vi "Type_1.vi"(7 "프런트패널 윈도우:동작":T2(ring)=enum."Default", 8 "에러 입력":errorcluster caption="에러 입력(에러 없음)", 11 "세부분류코드":string caption="확장자없는 파일 이름") -> (0 "error out":errorcluster)   [LabVIEW 2020]
uses:
  Support/Controls/Cmd_Mouse Popup.ctl
  Support/Controls/Clst_Query Info.ctl
  Support/Controls/Cmd_Read Query.ctl
  Support/Public/Polymorph/Data Class_2D Str.vi
  Support/Public/Polymorph/Array Dedup_1D Str.vi
  Support/Public/Polymorph/Cell Space_Table.vi
  <vilib>/addons/database/NI_Database_API.lvlib
panel:
  in  "탭 컨트롤":enum32{"검색", "등록", "CMC"}(tab)
  out "Calfunc":string[][](array[string])
  in  "Procedure 검색":T1(tab)
  in  "OPT_CODE 1":string(combo) caption="옵션 선택"
  in  "Func CbBox 1":string(combo) caption="Length_5"
  in  "Model List 1":i32(listbox) caption="모델 및 옵션 리스트"
  out "Load Proc 1":string[][](table) caption="등록된 교정 Procedure"
  in  "OPT_CODE 2":string(combo) caption="옵션 선택"
  in  "Func CbBox 2":string(combo) caption="Angle_1"
  in  "Model List 2":i32(listbox) caption="모델 및 옵션 리스트"
  out "Load Proc 2":string[][](table) caption="등록된 교정 Procedure"
  in  "OPT_CODE 3":string(combo) caption="옵션 선택"
  in  "Func CbBox 3":string(combo) caption="Magnification_1"
  in  "Model List 3":i32(listbox) caption="모델 및 옵션 리스트"
  out "Load Proc 3":string[][](table) caption="등록된 교정 Procedure"
  in  "OPT_CODE 4":string(combo) caption="옵션 선택"
  in  "Func CbBox 4":string(combo) caption="Right Angle_1"
  in  "Model List 4":i32(listbox) caption="모델 및 옵션 리스트"
  out "Load Proc 4":string[][](table) caption="등록된 교정 Procedure"
  in  "OPT_CODE 5":string(combo) caption="옵션 선택"
  in  "Func CbBox 5":string(combo) caption="AC Current Meter"
  in  "Model List 5":i32(listbox) caption="모델 및 옵션 리스트"
  out "Load Proc 5":string[][](table) caption="등록된 교정 Procedure"
  in  "OPT_CODE 6":string(combo) caption="옵션 선택"
  in  "Func CbBox 6":string(combo) caption="Frequency Meter"
  in  "Model List 6":i32(listbox) caption="모델 및 옵션 리스트"
  out "Load Proc 6":string[][](table) caption="등록된 교정 Procedure"
  in  "추가 버튼":bool
  out "소분류코드":string
  out "측정기명":string
  in  "단위":string(combo)
  in  "교정점 추가 버튼":bool
  in  "추가교정점":string
  out "Func_ext ?":bool
  out "배열":u32[](array[numeric])
  in  "Display 변경":bool
  in  "표시방식":string(combo)
  in  "Range":string(combo)
  in  "등록 버튼":bool
  in  "분해능 변경 버튼":bool
  in  "Proc":string[][](table) caption="등록할 교정 Procedure"
  in  "형식":string
  in  "옵션":string
  in  "분해능":string(combo)
  in  "교정기능":string(combo)
  out "CMC":string[][](table)
  # "항목정보"
  # "분해능 변경"
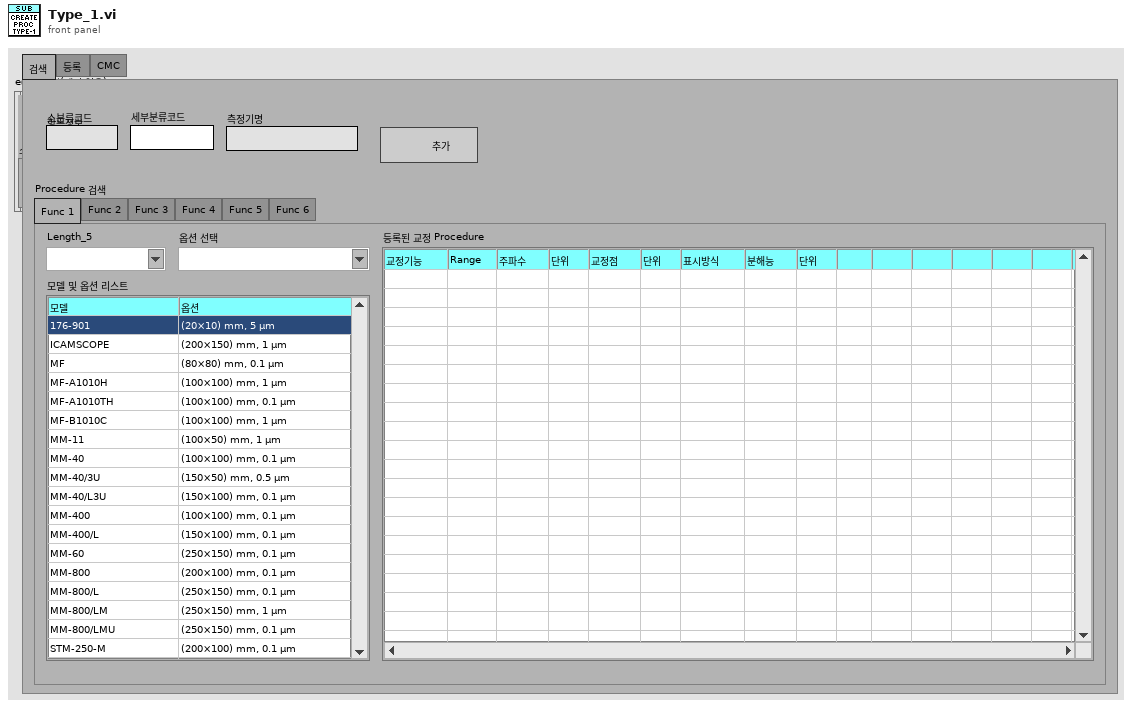
[diagram p1: front panel]
types:
  T1 = enum32{"Func 1", "Func 2", "Func 3", "Func 4", "Func 5", "Func 6"}
  T2 = enum32{"Invalid", "Default", "Floating", "Floating/Auto-Hide", "Modal"}
  T3 = typedef "Cmd_Mouse Popup.ctl" = enum16{"활성화", "메뉴선택"}
  T4 = cluster{"Shift":bool, "Ctrl":bool, "Alt":bool, "Cmd":bool, "Opt":bool}
  T5 = typedef "Clst_Query Info.ctl" = cluster{"사번":string, "등록번호":string, "업체명":string, "세부분류코드":string, "형식":string, "기기번호":string, "FUNC":string, "FUNC_EXT":string, "옵션":string, "추가문자열":string, "일자":string, "배열 1":string[], "배열 2":string[], "항목명":string, "문자열":string, "이름":string}
  T6 = typedef "Cmd_Read Query.ctl" = enum16{"교정자 이름 얻기", "인증교정자 얻기", "기술책임자 얻기", "기책부책 얻기", "등록번호 얻기", "등록정보 얻기", "업체정보 얻기", "교정일자(CAMAS) 얻기", "교정일자(CALSTD) 얻기", "교정환경 얻기", "교정절차서 목록 얻기", "교정절차서명 얻기", "교정절차 목록얻기", "교정절차 얻기", "PROC 교정절차 얻기", "PROC SPEC 얻기", "교정절차(Func별) 얻기", "교정절차(Func_ext별) 얻기", "기관코드 얻기", "교정기능(세부분류) 얻기", "교정기능(모델) 얻기", "교정기능 목록 얻기", "교정기능 명칭 얻기", "교정기능 항목명칭 얻기", "DB (사용기준기) 얻기", "DB (기준기이름) 얻기", "DB (기준기이름목록) 얻기", "DB (기준기목록) 얻기", "DB (기준기값) 얻기", "DB (CMC) 얻기", "DB (FUNC) 얻기", "DB (CALNAME) 얻기", "DB (STDNAME) 얻기", "DB (SPEC) 얻기", "모델(항목전체) 얻기", "모델(최대범위) 얻기", "모델(최소범위) 얻기", "모델(최대최소) 얻기", "모델(범위조건) 얻기", "모델(등록요청) 얻기", "모델(형식별) 얻기", "모델(조건별) 얻기", "모델(모델검색) 얻기", "세부분류 목록 얻기", "기준기등록리스트 얻기", "STD Cal Date Check", "DB등록일자 얻기", "적용항목 얻기", "기타정보 얻기", "기준기요청 얻기", "서버버전 얻기"}
  T7 = typedef "NI_Database_API.lvlib/Conn ObjectReference.ctl" = refnum<k1>
  T8 = typedef "LVRowAndColumnTypeDef.ctl" = cluster{"Row":i32, "Column":i32}
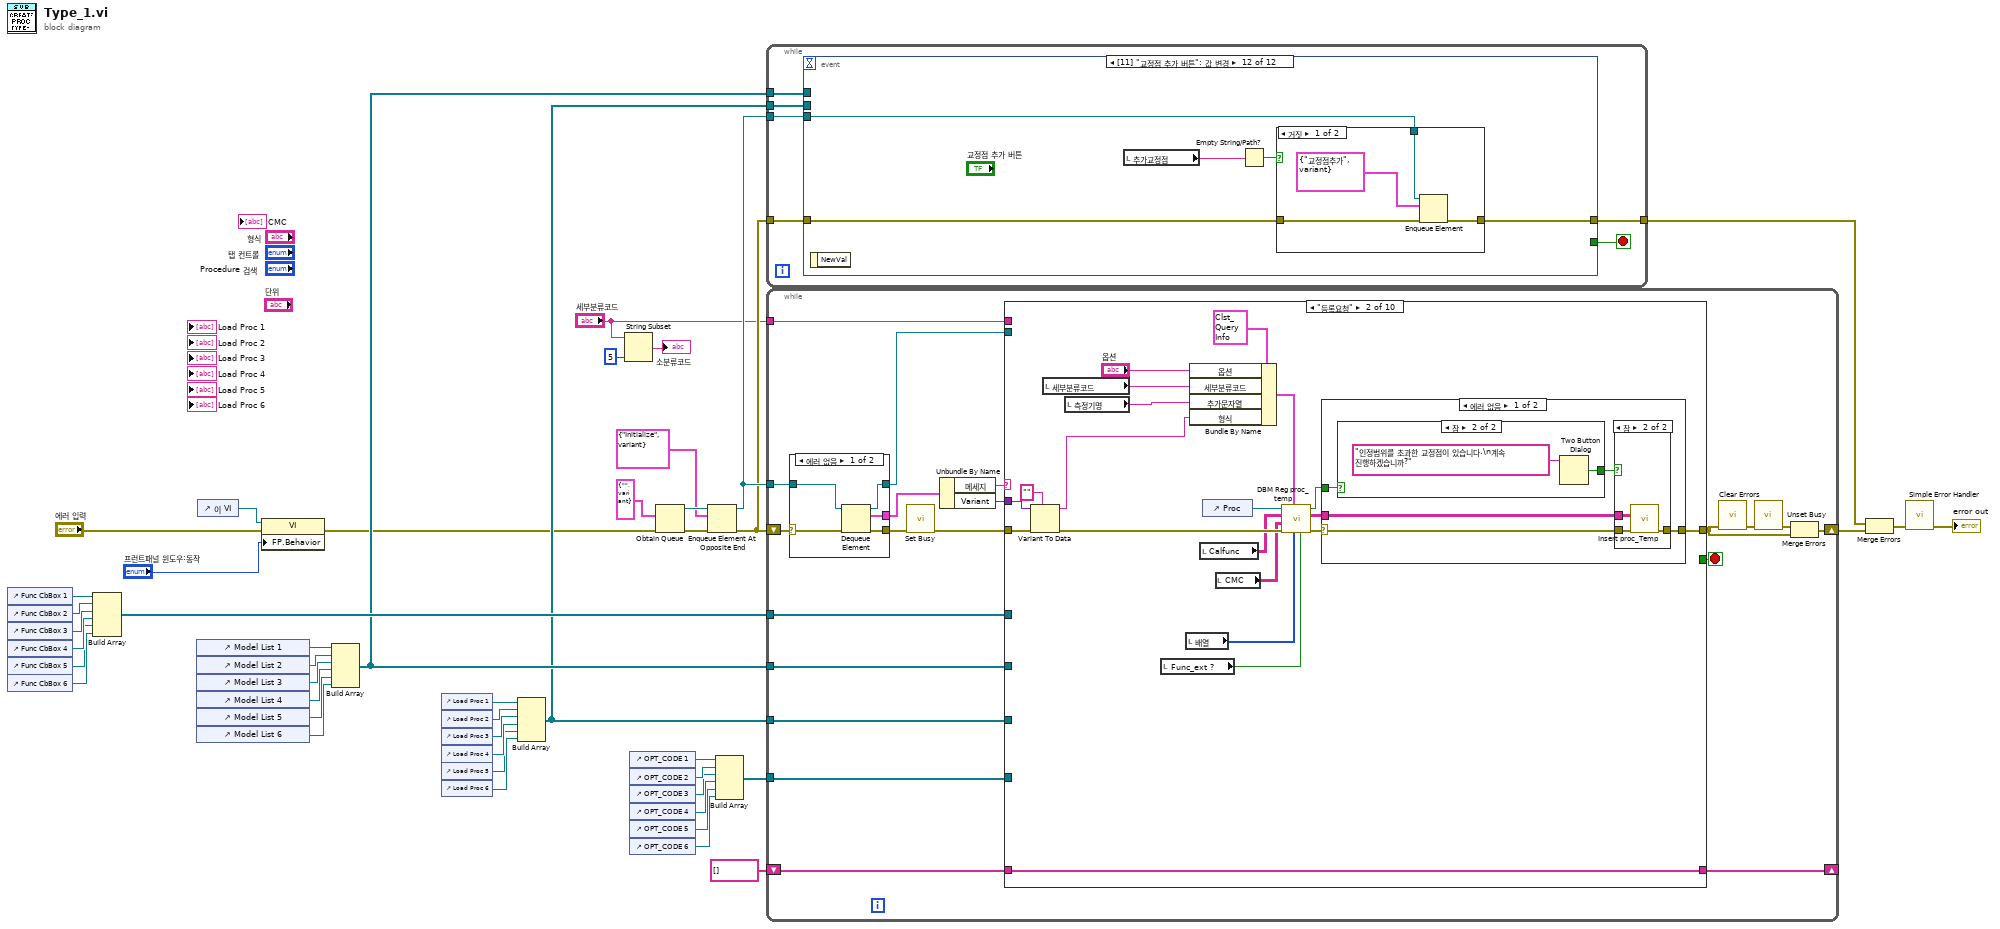
[diagram p0: block diagram]
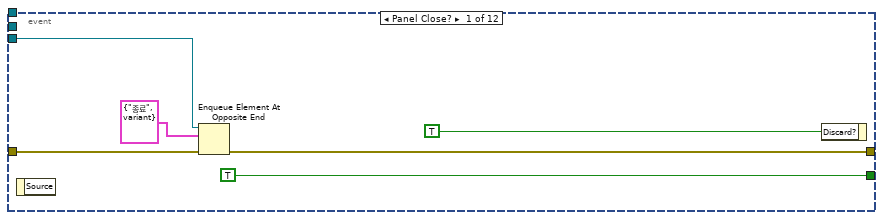
[diagram p2: hidden frame]
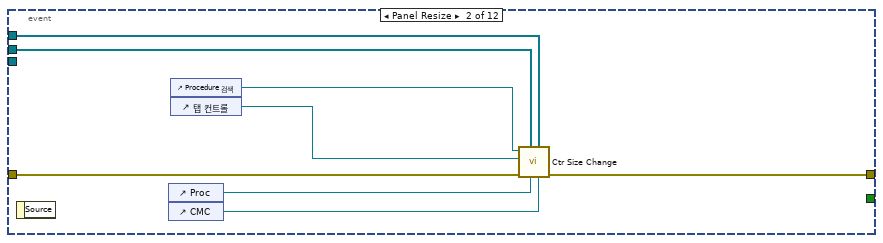
[diagram p3: hidden frame]
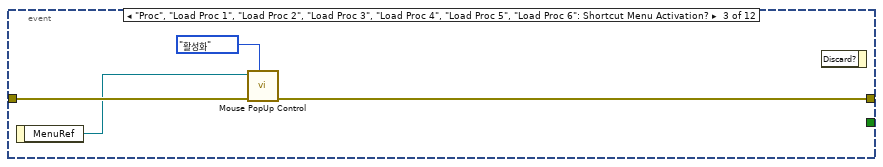
[diagram p4: hidden frame]
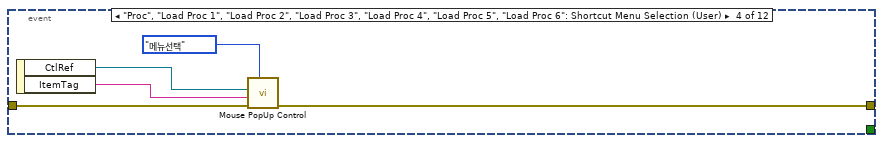
[diagram p5: hidden frame]
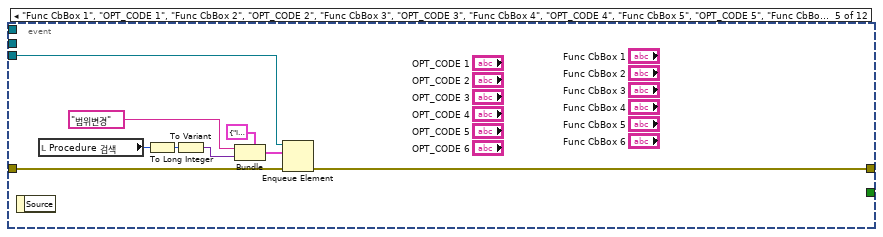
[diagram p6: hidden frame]
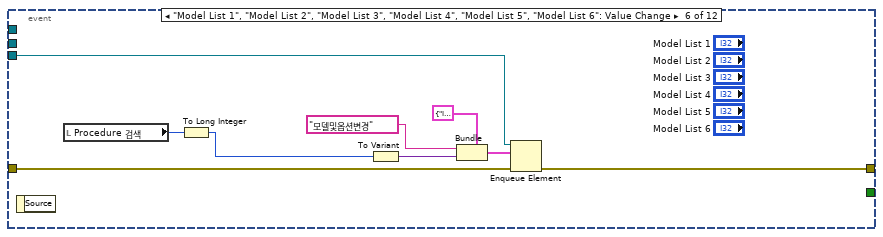
[diagram p7: hidden frame]
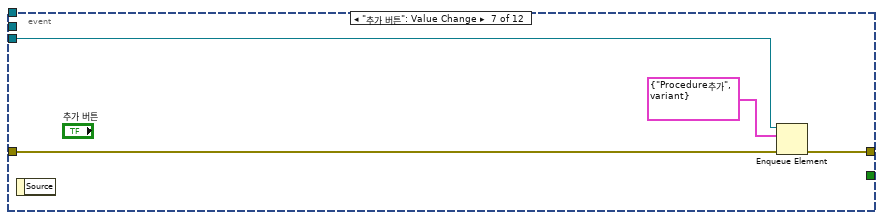
[diagram p8: hidden frame]
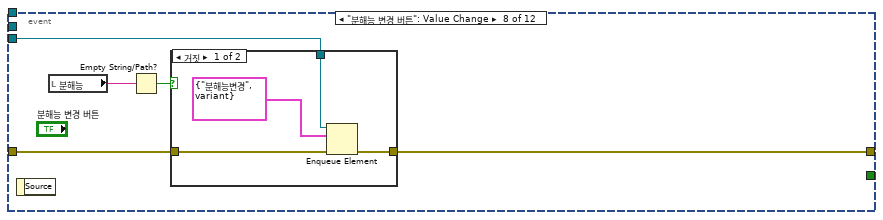
[diagram p9: hidden frame]
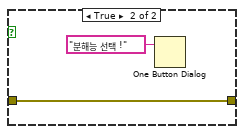
[diagram p10: hidden frame]
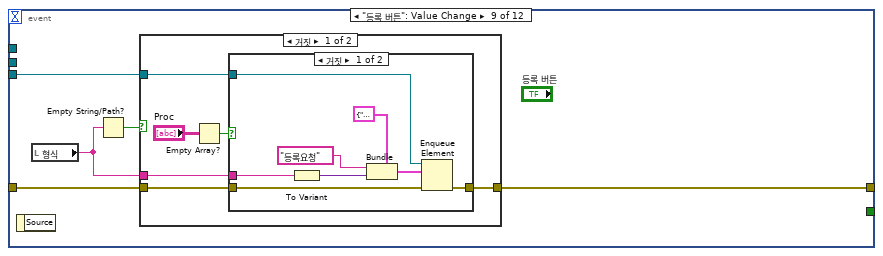
[diagram p11: hidden frame]
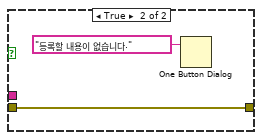
[diagram p12: hidden frame]
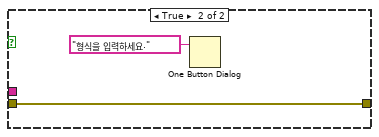
[diagram p13: hidden frame]
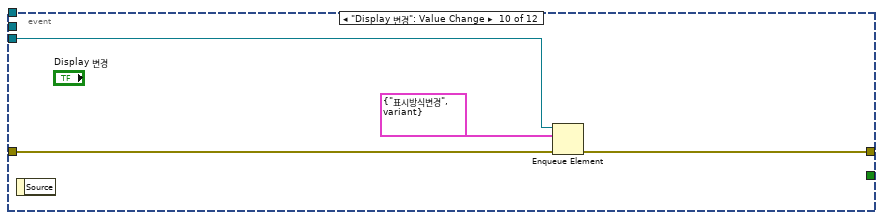
[diagram p14: hidden frame]
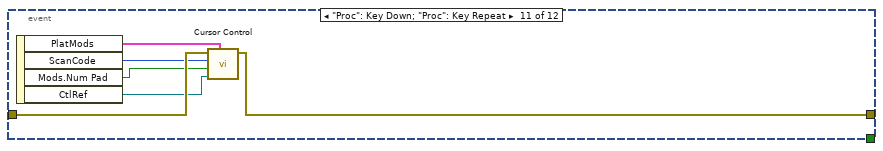
[diagram p15: hidden frame]
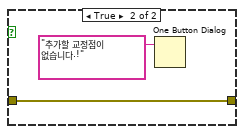
[diagram p16: hidden frame]
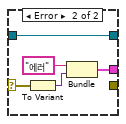
[diagram p17: hidden frame]
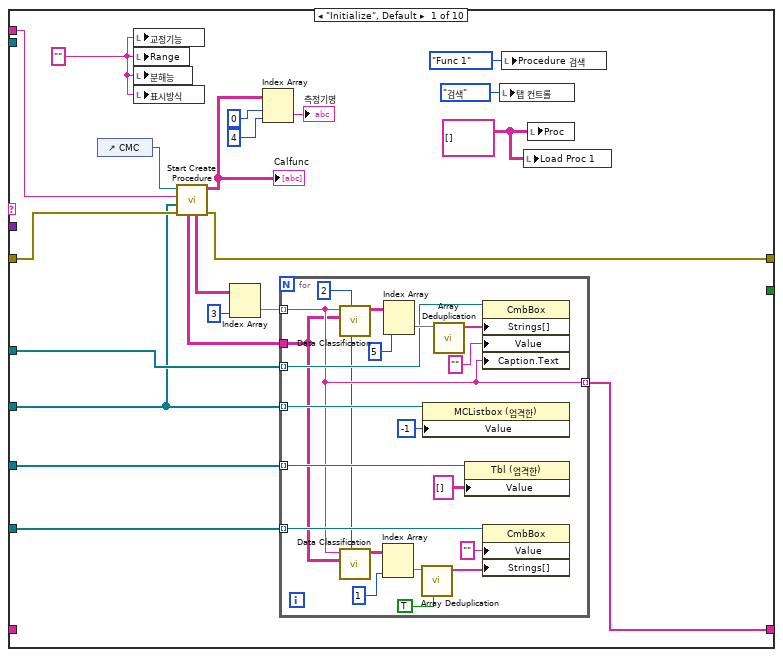
[diagram p18: hidden frame]
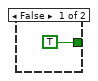
[diagram p19: hidden frame]
diagram:
  n1 = control-ref of="Func CbBox 1"() -> (w36:refnum<vi>)
  n2 = control-ref of="Func CbBox 2"() -> (w29:refnum<vi>)
  n3 = control-ref of="Func CbBox 3"() -> (w23:refnum<vi>)
  n4 = control-ref of="Func CbBox 4"() -> (w21:refnum<vi>)
  n5 = control-ref of="Func CbBox 5"() -> (w17:refnum<vi>)
  n6 = control-ref of="Func CbBox 6"() -> (w16:refnum<vi>)
  n7 = Build Array(w36, w29, w23, w21, w17, w16) -> (w35:refnum<vi>[])
  n8 = control-ref of="Model List 1"() -> (w33:refnum<vi>)
  n9 = control-ref of="Model List 2"() -> (w26:refnum<vi>)
  n10 = control-ref of="Model List 3"() -> (w25:refnum<vi>)
  n11 = control-ref of="Model List 4"() -> (w20:refnum<vi>)
  n12 = control-ref of="Model List 5"() -> (w15:refnum<vi>)
  n13 = control-ref of="Model List 6"() -> (w14:refnum<vi>)
  n14 = control-ref of="이 VI"() -> (w1:refnum<vi>)
  n15 = property class="VI"(reference=w1, error in="에러 입력", "FP.Behavior"="프런트패널 윈도우:동작") -> (error out=w6:errorcluster)  [unwired: 1 out]
  n16 = Build Array(w33, w26, w25, w20, w15, w14) -> (w9:refnum<vi>[])
  n17 = control-ref of="Load Proc 1"() -> (w32:refnum<vi>)
  n18 = control-ref of="Load Proc 2"() -> (w28:refnum<vi>)
  n19 = control-ref of="Load Proc 3"() -> (w24:refnum<vi>)
  n20 = control-ref of="Load Proc 4"() -> (w19:refnum<vi>)
  n21 = control-ref of="Load Proc 5"() -> (w13:refnum<vi>)
  n22 = control-ref of="Load Proc 6"() -> (w12:refnum<vi>)
  n23 = Build Array(w32, w28, w24, w19, w13, w12) -> (w8:refnum<vi>[])
  n24 = String Subset(string="세부분류코드", length (rest)=5 ("길이(나머지)")) -> (substring=→"소분류코드":string)  [unwired: 1 in]
  n25 = control-ref of="OPT_CODE 1"() -> (w31:refnum<vi>)
  n26 = control-ref of="OPT_CODE 2"() -> (w27:refnum<vi>)
  n27 = control-ref of="OPT_CODE 3"() -> (w22:refnum<vi>)
  n28 = control-ref of="OPT_CODE 4"() -> (w18:refnum<vi>)
  n29 = control-ref of="OPT_CODE 5"() -> (w11:refnum<vi>)
  n30 = control-ref of="OPT_CODE 6"() -> (w10:refnum<vi>)
  n31 = Obtain Queue(element data type=cluster{"메세지":string, "값":variant} {"메세지"="", "값"=variant} ("Message Cluster"), error in (no error)=w6) -> (queue out=w41:refnum<queue>, error out=w42:errorcluster)  [unwired: 3 in, 1 out]
  n32 = Enqueue Element At Opposite End(queue=w41, element=cluster{"메세지":string, "값":variant} {"메세지"="Initialize", "값"=variant} ("Message Cluster"), error in (no error)=w42) -> (queue out=w39:refnum<queue>, error out=w38:errorcluster)  [unwired: 1 in, 1 out]
  n33 = Build Array(w31, w27, w22, w18, w11, w10) -> (w30:refnum<vi>[])
  n34 = while {
    tunnel: w39 -> [w52]
    tunnel: w38 -> [w51]
    tunnel: [w50] -> w45
    tunnel: w9 -> [w48]
    tunnel: w8 -> [w47]
    stop <- w49 stop-if-true
    n35 = event shown="[11] \"교정점 추가 버튼\": 값 변경" {
      selector: _ -> [_ _ _ _ _ _ _ _ _ _ _ _]
      dyn-events: _ -> [_ _ _ _ _ _ _ _ _ _ _ _]
      timeout: _ -> [_ _ _ _ _ _ _ _ _ _ _ _]
      tunnel: w52 -> [w54 _ _ _ w83 w92 w96 w101 w111 w134 _ w143]
      tunnel: w51 -> [w56 w62 w70 w75 w78 w85 w95 w100 w113 w135 w141 w145]
      tunnel: [w55 w61 w69 w74 w84 w93 w97 w102 w112 w133 w137 w144] -> w50
      tunnel: [TRUE ("우선순위 메시지?") _ _ _ _ _ _ _ _ _ _ _] -> w49
      tunnel: w48 -> [_ w63 _ _ _ _ _ _ _ _ _ _]
      tunnel: w47 -> [_ w64 _ _ _ _ _ _ _ _ _ _]
      event Panel Close? {
        n36 = event-data() -> ()  [unwired: 1 in, 1 out]
        n37 = Enqueue Element At Opposite End(queue=w54, element=cluster{"메세지":string, "값":variant} {"메세지"="종료", "값"=variant} ("원소"), error in (no error)=w56) -> (error out=w55:errorcluster)  [unwired: 1 in, 2 out]
        n38 = event-data("Discard?"=TRUE ("버림?")) -> ()  [unwired: 1 in, 1 out]
      }
      event Panel Resize {
        n39 = event-data() -> ()  [unwired: 1 in, 1 out]
        n40 = control-ref of="Proc"() -> (w60:refnum<vi>)
        n41 = control-ref of="CMC"() -> (w59:refnum<vi>)
        n42 = control-ref of="Procedure 검색"() -> (w66:refnum<vi>)
        n43 = control-ref of="탭 컨트롤"() -> (w65:refnum<vi>)
        n44 = call "Ctr Size Change.vi"("CMC"=w59, "배열 2"=w63, "Proc"=w60, "배열"=w64, "error in (no error)"=w62, "탭 컨트롤"=w65, "TabControl 입력"=w66) -> ("error out"=w61:errorcluster)  [unwired: 4 in]
      }
      event "Proc", "Load Proc 1", "Load Proc 2", "Load Proc 3", "Load Proc 4", "Load Proc 5", "Load Proc 6": Shortcut Menu Activation? {
        n45 = event-data() -> ("MenuRef"=w67:refnum<k9>)  [unwired: 1 in]
        n46 = call "Mouse PopUp Control.vi"("type"=Cmd_Mouse_Popup."활성화", "error in"=w70, "메뉴 참조"=w67) -> ("error out"=w69:errorcluster)  [unwired: 8 in]
        n47 = event-data() -> ()  [unwired: 2 in, 1 out]
      }
      event "Proc", "Load Proc 1", "Load Proc 2", "Load Proc 3", "Load Proc 4", "Load Proc 5", "Load Proc 6": Shortcut Menu Selection (User) {
        n48 = event-data() -> ("CtlRef"=w71:refnum<vi>, "ItemTag"=w72:string)  [unwired: 1 in]
        n49 = call "Mouse PopUp Control.vi"("type"=Cmd_Mouse_Popup."메뉴선택", "error in"=w75, "아이템 태그"=w72, "Tbl 참조 번호"=w71) -> ("error out"=w74:errorcluster)  [unwired: 7 in]
      }
      event "Func CbBox 1", "OPT_CODE 1", "Func CbBox 2", "OPT_CODE 2", "Func CbBox 3", "OPT_CODE 3", "Func CbBox 4", "OPT_CODE 4", "Func CbBox 5", "OPT_CODE 5", "Func CbBox 6", "OPT_CODE 6": Value Change {
        n50 = event-data() -> ()  [unwired: 1 in, 1 out]
        n51 = local read "Procedure 검색"() -> (w77:T1)
        n52 = To Long Integer(number=w77) -> (32bit integer=w76:i32)
        n53 = To Variant(anything=w76) -> (Variant=w80:variant)
        n54 = Bundle(cluster=cluster{"메세지":string, "값":variant} {"메세지"="Initialize", "값"=variant} ("Message Cluster"), "메세지"="범위변경", "값"=w80) -> (w79:cluster{"메세지":string, "값":variant})
        n55 = Enqueue Element(queue=w83, element=w79, error in (no error)=w78) -> (error out=w84:errorcluster)  [unwired: 1 in, 2 out]
      }
      event "Model List 1", "Model List 2", "Model List 3", "Model List 4", "Model List 5", "Model List 6": Value Change {
        n56 = event-data() -> ()  [unwired: 1 in, 1 out]
        n57 = local read "Procedure 검색"() -> (w87:T1)
        n58 = To Long Integer(number=w87) -> (32bit integer=w86:i32)
        n59 = To Variant(anything=w86) -> (Variant=w89:variant)
        n60 = Bundle(cluster=cluster{"메세지":string, "값":variant} {"메세지"="Initialize", "값"=variant} ("Message Cluster"), "메세지"="모델및옵션변경", "값"=w89) -> (w88:cluster{"메세지":string, "값":variant})
        n61 = Enqueue Element(queue=w92, element=w88, error in (no error)=w85) -> (error out=w93:errorcluster)  [unwired: 1 in, 2 out]
      }
      event "추가 버튼": Value Change {
        n62 = event-data() -> ()  [unwired: 1 in, 1 out]
        n63 = Enqueue Element(queue=w96, element=cluster{"메세지":string, "값":variant} {"메세지"="Procedure추가", "값"=variant} ("Message Cluster"), error in (no error)=w95) -> (error out=w97:errorcluster)  [unwired: 1 in, 2 out]
      }
      event "분해능 변경 버튼": Value Change {
        n64 = event-data() -> ()  [unwired: 1 in, 1 out]
        n65 = local read "분해능"() -> (w99:string)
        n66 = Empty String/Path?(string/path=w99) -> (empty?=w98:bool)
        n67 = case shown="거짓" w98 {
          tunnel: [w106 w108] -> w102
          tunnel: w101 -> [w105 _]
          tunnel: w100 -> [w104 w108]
          frame False {
            n68 = Enqueue Element(queue=w105, element=cluster{"메세지":string, "값":variant} {"메세지"="분해능변경", "값"=variant} ("Message Cluster"), error in (no error)=w104) -> (error out=w106:errorcluster)  [unwired: 1 in, 2 out]
          }
          frame True {
            n69 = One Button Dialog(message="분해능 선택 !" ("메시지")) -> ()  [unwired: 1 in, 1 out]
          }
        }
      }
      event "등록 버튼": Value Change {
        n70 = event-data() -> ()  [unwired: 1 in, 1 out]
        n71 = local read "형식"() -> (w109:string)
        n72 = Empty String/Path?(string/path=w109) -> (empty?=w110:bool)
        n73 = case shown="거짓" w110 {
          tunnel: w113 -> [w119 w131]
          tunnel: [w118 w131] -> w112
          tunnel: w111 -> [w117 _]
          tunnel: w109 -> [w116 _]
          frame False {
            n74 = Empty Array?(array="Proc") -> (empty?=w114:bool)
            n75 = case shown="거짓" w114 {
              tunnel: w119 -> [w127 w129]
              tunnel: [w126 w129] -> w118
              tunnel: w117 -> [w125 _]
              tunnel: w116 -> [w122 _]
              frame False {
                n76 = To Variant(anything=w122) -> (Variant=w121:variant)
                n77 = Bundle(cluster=cluster{"메세지":string, "값":variant} {"메세지"="", "값"=variant} ("원소"), "메세지"="등록요청", "값"=w121) -> (w123:cluster{"메세지":string, "값":variant})
                n78 = Enqueue Element(queue=w125, element=w123, error in (no error)=w127) -> (error out=w126:errorcluster)  [unwired: 1 in, 2 out]
              }
              frame True {
                n79 = One Button Dialog(message="등록할 내용이 없습니다." ("메시지")) -> ()  [unwired: 1 in, 1 out]
              }
            }
          }
          frame True {
            n80 = One Button Dialog(message="형식을 입력하세요." ("메시지")) -> ()  [unwired: 1 in, 1 out]
          }
        }
      }
      event "Display 변경": Value Change {
        n81 = event-data() -> ()  [unwired: 1 in, 1 out]
        n82 = Enqueue Element(queue=w134, element=cluster{"메세지":string, "값":variant} {"메세지"="표시방식변경", "값"=variant} ("Message Cluster"), error in (no error)=w135) -> (error out=w133:errorcluster)  [unwired: 1 in, 2 out]
      }
      event "Proc": Key Down; "Proc": Key Repeat {
        n83 = event-data() -> ("PlatMods"=w136:T4, "ScanCode"=w140:i16, "Mods.Num Pad"=w139:bool, "CtlRef"=w138:refnum<vi>)  [unwired: 1 in]
        n84 = call "Cursor Control.vi"("플랫폼 조합키"=w136, "참조"=w138, "Num Pad"=w139, "ScanCode"=w140, "error in"=w141) -> ("error out"=w137:errorcluster)  [unwired: 5 in, 1 out]
      }
      event "교정점 추가 버튼": Value Change {
        n85 = event-data() -> ()  [unwired: 1 in, 1 out]
        n86 = local read "추가교정점"() -> (w142:string)
        n87 = Empty String/Path?(string/path=w142) -> (empty?=w146:bool)
        n88 = case shown="거짓" w146 {
          tunnel: [w150 w152] -> w144
          tunnel: w143 -> [w149 _]
          tunnel: w145 -> [w148 w152]
          frame False {
            n89 = Enqueue Element(queue=w149, element=cluster{"메세지":string, "값":variant} {"메세지"="교정점추가", "값"=variant} ("Message Cluster"), error in (no error)=w148) -> (error out=w150:errorcluster)  [unwired: 1 in, 2 out]
          }
          frame True {
            n90 = One Button Dialog(message="추가할 교정점이  없습니다.!" ("메시지")) -> ()  [unwired: 1 in, 1 out]
          }
        }
      }
    }
  }
  n91 = while {
    tunnel: w39 -> [w171]
    shift-right: [w161] -> w46
    shift-left: w38 -> [w167]
    tunnel: w35 -> [w165]
    tunnel: w9 -> [w158]
    shift-right: [w157] -> _
    shift-left: string[] [] -> [w156]
    tunnel: w8 -> [w155]
    tunnel: w30 -> [w154]
    tunnel: "세부분류코드" -> [w153]
    stop <- w172 stop-if-true
    n92 = case shown="에러 없음" w167 {
      selector: w167 -> [w173 w178]
      tunnel: w171 -> [w177 w182]
      tunnel: [w176 _] -> w164
      tunnel: [w174 w182] -> w170
      tunnel: [w175 w181] -> w166
      frame No Error {
        n93 = Dequeue Element(queue=w177, error in (no error)=w173) -> (queue out=w174:refnum<queue>, element=w175:cluster{"메세지":string, "값":variant}, error out=w176:errorcluster)  [unwired: 1 in, 1 out]
      }
      frame Error {
        n94 = To Variant(anything=w178) -> (Variant=w179:variant)
        n95 = Bundle("에러", "Variant"=w179) -> (w181:cluster{string, "Variant":variant})  [unwired: 1 in]
      }
    }
    n96 = call <vilib>:"Set Busy.vi"("error in (no error)"=w164) -> ("error out"=w163:errorcluster)  [unwired: 9 in, 1 out]
    n97 = Unbundle By Name(w166) -> ("메세지"=w168:string, "Variant"=w169:variant)
    n98 = case shown="\"등록요청\"" w168 {
      tunnel: w163 -> [w203 w242 w279 w314 w324 w335 w353 w373 w380 w386]
      tunnel: [w200 w229 w276 w311 w322 w333 w353 w373 w380 w383] -> w159
      tunnel: w170 -> [_ _ _ _ _ _ _ _ _ _]
      tunnel: w169 -> [_ w241 w278 w313 _ _ _ _ _ w384]
      tunnel: [_ _ _ _ _ _ _ _ TRUE _] -> w172
      tunnel: w165 -> [w196 _ w265 _ _ _ _ _ _ _]
      tunnel: w158 -> [w195 _ w264 w297 _ _ _ _ _ _]
      tunnel: w156 -> [_ w234 w263 w292 w321 w336 w348 w372 w378 w381]
      tunnel: [w199 w234 w263 w292 w321 w336 w348 w372 w378 w381] -> w157
      tunnel: w155 -> [w198 _ _ w294 w320 _ _ _ _ _]
      tunnel: w154 -> [w197 _ _ w289 _ _ _ _ _ _]
      tunnel: w153 -> [w185 _ _ _ _ _ _ _ _ _]
      frame "Initialize", Default {
        w193 = ""
        w201 = string[][] [] ("Proc")
        n99 = control-ref of="CMC"() -> (w186:refnum<vi>)
        n100 = local write "교정기능"(w193) -> ()
        n101 = local write "Range"(w193) -> ()
        n102 = local write "분해능"(w193) -> ()
        n103 = local write "표시방식"(w193) -> ()
        n104 = call "Start Create Procedure.vi"("에러 입력(에러 없음)"=w203, "Model List"=w195, "세부분류코드"=w185, "CMC"=w186) -> ("에러 출력"=w200:errorcluster, "Calfunc"=w184:string[][], "Data"=w192:string[][], "모델정보 배열"=w183:string[][])  [unwired: 2 in, 2 out]
        "Calfunc" <- w184
        n105 = Index Array(array=w192, index (col)=3 ("비활성화된 인덱스 (열)")) -> (element=w190:string[])  [unwired: 1 in]
        n106 = Index Array(array=w184, index (row)=0 ("인덱스 (열)"), index (col)=4 ("비활성화된 인덱스 (열)")) -> (element=→"측정기명":string)
        n107 = for {
          tunnel: w190 -> [w211] mode=indexing
          tunnel: w183 -> [w210]
          tunnel: w196 -> [w220] mode=indexing
          tunnel: [w211] -> w199 mode=indexing
          tunnel: w195 -> [w217] mode=indexing
          tunnel: w198 -> [w215] mode=indexing
          tunnel: w197 -> [w214] mode=indexing
          w209 = 2 ("인덱스")
          n108 = call-poly "Data Classification.vi"("인덱스"=w209, "DATA 입력"=w210, "검색 문자열"=w211) -> ("DATA 출력"=w223:string[][])  [unwired: 4 in, 4 out]
          n109 = call-poly "Data Classification.vi"("인덱스"=w209, "DATA 입력"=w210, "검색 문자열"=w211) -> ("DATA 출력"=w208:string[][])  [unwired: 4 in, 4 out]
          n110 = Index Array(array=w208, index (col)=1 ("비활성화된 인덱스 (열)")) -> (element=w206:string[])  [unwired: 1 in]
          n111 = Index Array(array=w223, index (col)=5 ("비활성화된 인덱스 (열)")) -> (element=w222:string[])  [unwired: 1 in]
          n112 = call-poly "Array Deduplication.vi"("정렬?"=TRUE, "배열 in"=w206) -> ("배열 out"=w205:string[])  [unwired: 8 in, 1 out]
          n113 = property class="MCListbox (엄격한)"(reference=w217, "Value"=-1 ("값")) -> ()  [unwired: 1 in, 2 out]
          n114 = call-poly "Array Deduplication.vi"("배열 in"=w222) -> ("배열 out"=w219:string[])  [unwired: 9 in, 1 out]
          n115 = property class="Tbl (엄격한)"(reference=w215, "Value"=string[][] [] ("값")) -> ()  [unwired: 1 in, 2 out]
          n116 = property class="CmbBox"(reference=w220, "Strings[]"=w219, "Value"="" ("값"), "Caption.Text"=w211) -> ()  [unwired: 1 in, 2 out]
          n117 = property class="CmbBox"(reference=w214, "Value"="" ("값"), "Strings[]"=w205) -> ()  [unwired: 1 in, 2 out]
        }
        n118 = local write "탭 컨트롤"(enum32{"검색", "등록", "CMC"}."검색" ("탭 컨트롤")) -> ()
        n119 = local write "Procedure 검색"(T1."Func 1" ("Procedure 검색")) -> ()
        n120 = local write "Load Proc 1"(w201) -> ()
        n121 = local write "Proc"(w201) -> ()
      }
      frame "등록요청" {
        n122 = Variant To Data(error in=w242, type="", Variant=w241) -> (data=w224:string)  [unwired: 1 out]
        n123 = local read "세부분류코드"() -> (w237:string)
        n124 = local read "측정기명"() -> (w236:string)
        n125 = local read "Func_ext ?"() -> (w231:bool)
        n126 = local read "배열"() -> (w232:u32[])
        n127 = Bundle By Name(cluster=T5 {"사번"="", "등록번호"="", "업체명"="", "세부분류코드"="", "형식"="", "기기번호"="", "FUNC"="", "FUNC_EXT"="", "옵션"="", "추가문자열"="", "일자"="", "배열 1"=[], "배열 2"=[], "항목명"="", "문자열"="", "이름"=""} ("Query info"), "옵션"="옵션", "세부분류코드"=w237, "추가문자열"=w236, "형식"=w224) -> (w226:T5)
        n128 = local read "Calfunc"() -> (w233:string[][])
        n129 = control-ref of="Proc"() -> (w225:refnum<vi>)
        n130 = local read "CMC"() -> (w235:string[][])
        n131 = call "DBM Reg proc_temp.vi"("Calfunc ?"=w231, "배열"=w232, "Query info"=w226, "에러 입력"=w242, "CMC"=w235, "calfunc"=w233, "Proc 참조 in"=w225) -> ("에러 출력"=w230:errorcluster, "배열출력"=w228:string[][], "에러?"=w227:bool)  [unwired: 2 in]
        n132 = case shown="에러 없음" w230 {
          selector: w230 -> [w243 w255]
          tunnel: w227 -> [w247 _]
          tunnel: [w246 w255] -> w229
          tunnel: w228 -> [w245 _]
          frame No Error {
            n133 = case shown="참" w247 {
              tunnel: [TRUE ("T button?") w249] -> w244
              frame False {
              }
              frame True {
                n134 = Two Button Dialog(message="인정범위를 초과한 교정점이 있습니다.\n계속 진행하겠습니까?" ("메시지")) -> (T button?=w249:bool)  [unwired: 2 in]
              }
            }
            n135 = case shown="참" w244 {
              tunnel: [w251 w254] -> w246
              tunnel: w243 -> [w251 w253]
              tunnel: w245 -> [_ w252]
              frame False {
              }
              frame True {
                n136 = call "Insert proc_Temp.vi"("에러 입력(에러 없음)"=w253, "Proc 입력"=w252) -> ("에러 출력"=w254:errorcluster)  [unwired: 9 in]
              }
            }
          }
          frame Error {
          }
        }
      }
      frame "범위변경" {
        n137 = Variant To Data(error in=w279, type=0, Variant=w278) -> (data=w262:i32, error out=w267:errorcluster)
        n138 = Index Array(array=w265, index=w262) -> (element=w261:refnum<vi>)
        n139 = Index Array(array=w264, index=w262) -> (element=w258:refnum<vi>)
        n140 = Index Array(array=w263, index=w262) -> (element=w259:string)
        n141 = property class="CmbBox"(reference=w261) -> ("Value"=w260:string)  [unwired: 1 in, 2 out]
        n142 = local read "OPT_CODE 1"() -> (w257:string)
        n143 = call "DB Open.vi"("에러 입력"=w267) -> ("에러 출력"=w275:errorcluster, "참조 번호 출력"=w272:T7)  [unwired: 9 in]
        n144 = Bundle By Name(cluster=T5 {"사번"="", "등록번호"="", "업체명"="", "세부분류코드"="", "형식"="", "기기번호"="", "FUNC"="", "FUNC_EXT"="", "옵션"="", "추가문자열"="", "일자"="", "배열 1"=[], "배열 2"=[], "항목명"="", "문자열"="", "이름"=""} ("Query info"), "옵션"=w257, "추가문자열"=w260, "FUNC"=w259) -> (w268:T5)
        n145 = call "DB Read Queries.vi"("Query info"=w268, "Query Command"=Cmd_Read_Query."모델(범위조건) 얻기", "에러 입력(에러 없음)"=w275, "참조 번호 입력"=w272) -> ("에러 출력"=w274:errorcluster, "Data"=w273:string[][], "참조 번호 출력"=w271:T7)  [unwired: 3 in, 2 out]
        n146 = call <vilib>:"DB Tools Close Connection.vi"("error in (no error)"=w274, "connection reference"=w271) -> ("error out"=w277:errorcluster)  [unwired: 5 in]
        n147 = property on="프로퍼티 노드" class="MCListbox (엄격한)"(reference=w258, error in=w277, "ItemNames"=w273, "Value"=-1 ("값")) -> (error out=w276:errorcluster)  [unwired: 1 out]
      }
      frame "모델및옵션변경" {
        n148 = Variant To Data(error in=w314, type=0, Variant=w313) -> (data=w288:i32, error out=w295:errorcluster)
        n149 = Index Array(array=w289, index=w288) -> (element=w287:refnum<vi>)
        n150 = Index Array(array=w294, index=w288) -> (element=w293:refnum<vi>)
        n151 = Index Array(array=w292, index=w288) -> (element=w283:string)
        n152 = Index Array(array=w297, index=w288) -> (element=w296:refnum<vi>)
        n153 = property on="프로퍼티 노드" class="MCListbox (엄격한)"(reference=w296) -> ("ItemNames"=w298:string[][], "Value"=w299:i32)  [unwired: 1 in, 2 out]
        n154 = property on="프로퍼티 노드" class="CmbBox"(reference=w287) -> ("Value"=w286:string)  [unwired: 1 in, 2 out]
        n155 = local read "세부분류코드"() -> (w304:string)
        n156 = Index Array(array=w298, index (row)=w299, index (col)=0 ("비활성화된 인덱스 (열)")) -> (element=w290:string)
        n157 = Bundle By Name(cluster=T5 {"사번"="", "등록번호"="", "업체명"="", "세부분류코드"="", "형식"="", "기기번호"="", "FUNC"="", "FUNC_EXT"="", "옵션"="", "추가문자열"="", "일자"="", "배열 1"=[], "배열 2"=[], "항목명"="", "문자열"="", "이름"=""} ("Query info"), "세부분류코드"=w304, "FUNC"=w283, "형식"=w290, "옵션"=w286) -> (w303:T5)
        n158 = call "DB Open.vi"("에러 입력"=w295) -> ("에러 출력"=w310:errorcluster, "참조 번호 출력"=w308:T7)  [unwired: 9 in]
        n159 = call "DB Read Queries.vi"("Query info"=w303, "Query Command"=Cmd_Read_Query."교정절차(Func별) 얻기", "에러 입력(에러 없음)"=w310, "참조 번호 입력"=w308) -> ("에러 출력"=w309:errorcluster, "Data"=w302:string[][], "참조 번호 출력"=w307:T7)  [unwired: 3 in, 2 out]
        n160 = local read "Calfunc"() -> (w282:string[][])
        n161 = call <vilib>:"DB Tools Close Connection.vi"("error in (no error)"=w309, "connection reference"=w307) -> ("error out"=w284:errorcluster)  [unwired: 5 in]
        n162 = call "Condition Filter.vi"("Cal func in"=w282, "컬럼명"="func\nc2_val\nc3_val\nc4_val\ncal_val\ncal_unit\ndisp_sys\nresol\nresol_unit" ("SQL query"), "error in (no error)"=w284, "Cal Proc in"=w302) -> ("error out"=w285:errorcluster, "배열"=→"배열":u32[], "Func_ext ?"=→"Func_ext ?":bool, "Cal Proc out"=w301:string[][])  [unwired: 4 in]
        n163 = call-poly "Cell Spacing.vi"("error in"=w285, "Data in"=w301, "테이블 참조 in"=w293) -> ("error out"=w311:errorcluster)  [unwired: 6 in, 2 out]
      }
      frame "Procedure추가" {
        n164 = for {
          tunnel: w320 -> [w329] mode=indexing
          tunnel: [w328] -> w319 mode=concatenating if=w326
          n165 = property class="Tbl (엄격한)"(reference=w329) -> ("Value"=w328:string[][])  [unwired: 1 in, 2 out]
          n166 = Empty Array?(array=w328) -> (empty?=w327:bool)
          n167 = Not(x=w327) -> (.not. x?=w326:bool)
        }
        n168 = local write "탭 컨트롤"(enum32{"검색", "등록", "CMC"}."등록" ("탭 컨트롤")) -> ()
        n169 = control-ref of="Proc"() -> (w315:refnum<vi>)
        n170 = call-poly "Cell Spacing.vi"("error in"=w324, "Data in"=w319, "테이블 참조 in"=w315) -> ("error out"=w318:errorcluster)  [unwired: 6 in, 2 out]
        n171 = Index Array(array=w319, index (col)=1 ("비활성화된 인덱스 (열)")) -> (element=w317:string[])  [unwired: 1 in]
        n172 = call-poly "Array Deduplication.vi"("error in (no error)"=w318, "배열 in"=w317) -> ("배열 out"=w316:string[])  [unwired: 8 in, 1 out]
        n173 = property on="Range" class="CmbBox"(error in=w318, "Strings[]"=w316) -> (error out=w322:errorcluster)  [unwired: 1 in, 1 out]
      }
      frame "교정점추가" {
        n174 = property on="Proc" class="Tbl (엄격한)"(error in=w335) -> (error out=w333:errorcluster, "Value"=w332:string[][], "Selection Start"=w334:T8, "Column Headers[]"=w330:string[])  [unwired: 1 in, 1 out]
        n175 = Unbundle(w334) -> ("Row"=w331:i32)  [unwired: 1 out]
        n176 = case shown="기본" w331 {
          selector: w331 -> [_ w340]
          tunnel: w332 -> [_ w341]
          tunnel: w330 -> [_ w338]
          frame 0 {
          }
          frame Default {
            n177 = Decrement(x=w340) -> (x-1=w344:i32)
            n178 = Index Array(array=w341, index (row)=w344) -> (element=w342:string[])  [unwired: 1 in]
            n179 = Search 1D Array(1D array=w338, element="교정점" ("원소")) -> (index of element=w346:i32)  [unwired: 1 in]
            n180 = Replace Array Subset(array=w342, new element="추가교정점", index=w346) -> (w343:string[])
            n181 = Insert Into Array(array=w341, index (row)=w340, new element=w343) -> (w337:string[][])  [unwired: 1 in]
            n182 = local write "Proc"(w337) -> ()
          }
        }
      }
      frame "분해능변경" {
        n183 = local read "Proc"() -> (w352:string[][])
        n184 = for {
          tunnel: w352 -> [w361] mode=indexing
          tunnel: "분해능" -> [w363]
          tunnel: [w362] -> w350 mode=indexing
          tunnel: "교정기능" -> [w360]
          tunnel: "Range" -> [w357]
          n185 = Index Array(array=w361) -> (element #1=w359:string, element #2=w358:string)  [unwired: 2 in]
          n186 = Equal?(x=w359, y=w360) -> (x = y?=w356:bool)
          n187 = Equal?(x=w358, y=w357) -> (x = y?=w355:bool)
          n188 = Compound Arithmetic op=AND(w356, w355) -> (w354:bool)
          n189 = case shown="참" w354 {
            tunnel: w363 -> [_ w368]
            tunnel: [w364 w367] -> w362
            tunnel: w361 -> [w364 w365]
            frame False {
            }
            frame True {
              n190 = Replace Array Subset(array=w365, new element=w368, index=7 ("인덱스")) -> (w367:string[])
            }
          }
        }
        n191 = local write "Proc"(w350) -> ()
      }
      frame "표시방식변경" {
        n192 = local read "Proc"() -> (w371:string[][])
        n193 = for {
          tunnel: w371 -> [w377] mode=indexing
          tunnel: "표시방식" -> [w376]
          tunnel: [w374] -> w369 mode=indexing
          n194 = Replace Array Subset(array=w377, new element=w376, index=6 ("인덱스")) -> (w374:string[])
        }
        n195 = local write "Proc"(w369) -> ()
      }
      frame "종료" {
      }
      frame "에러" {
        n196 = Variant To Data(error in=w386, type=errorcluster {"status"=FALSE, "code"=0, "source"=""} ("에러 출력"), Variant=w384) -> (data=w382:errorcluster, error out=w383:errorcluster)
        n197 = call <vilib>:"Simple Error Handler.vi"("error in (no error)"=w382) -> ()  [unwired: 4 in, 5 out]
      }
    }
    n198 = call <vilib>:"Clear Errors.vi"("error in (no error)"=w159) -> ("error out"=w162:errorcluster)  [unwired: 5 in, 1 out]
    n199 = call <vilib>:"Unset Busy.vi"("error in (no error)"=w162) -> ("error out"=w160:errorcluster)  [unwired: 10 in]
    n200 = Merge Errors(w160, w159) -> (w161:errorcluster)
  }
  n201 = Merge Errors(w45, w46) -> (w44:errorcluster)
  n202 = call <vilib>:"Simple Error Handler.vi"("error in (no error)"=w44) -> ("error out"=→"error out":errorcluster)  [unwired: 4 in, 4 out]
